vi "SetFs.vi"(8 "error in (no error)":errorcluster, 9 "Fs":dbl format="%#_6pHz", 10 "Port":string(combo), 11 "reference in":refnum<class "mmWave instrument.lvclass">) -> (0 "error out":errorcluster, 3 "reference out":refnum<class "mmWave instrument.lvclass">)   [LabVIEW 2019, in "mmWave instrument.lvclass"]
doc: "Set sampling frequency for port"
uses:
  mmWave instrument.lvclass
  mmWave HW Control/HW custom error.ctl
  mmWave HW Control/mmWave HW Control.lvlib
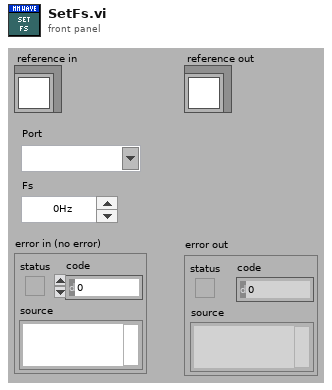
[diagram p1: front panel]
types:
  T1 = typedef "mmWave HW Control.lvlib/HW custom error.ctl" = u16
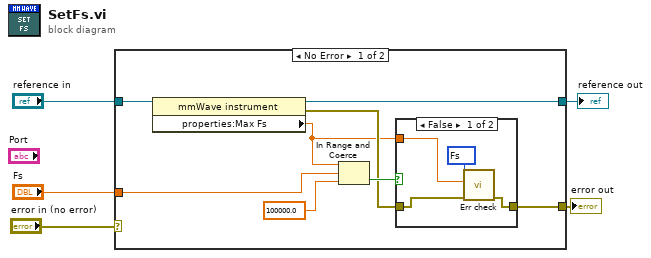
[diagram p0: block diagram]
diagram:
  n1 = case shown="No Error" "error in (no error)" {
    selector: "error in (no error)" -> [_ w20]
    tunnel: [w8 w20] -> w4
    tunnel: [w12 w19] -> w2
    tunnel: "reference in" -> [w13 w19]
    tunnel: "Fs" -> [w11 _]
    frame No Error {
      n2 = property class="mmWave instrument"(reference=w13) -> (reference out=w12:refnum<class "mmWave instrument.lvclass">, error out=w7:errorcluster, "properties:Max Fs"=w6:dbl)  [unwired: 1 in]
      n3 = In Range and Coerce(upper limit=w6, x=w11, lower limit=100000.0) -> (In Range?=w9:bool)  [unwired: 1 out]
      n4 = case shown="False" w9 {
        tunnel: [w14 w18] -> w8
        tunnel: w7 -> [w15 w18]
        tunnel: w6 -> [w17 _]
        frame False {
          w16 = T1 10003 items=["TX list"=10000, "TX length"=10001, "RX length"=10002, "Fs"=10003] ("HW custom err")
          n5 = call "Err check.vi"("error in"=w15, "Variant Control"=w17, "HW custom err"=w16) -> ("error out"=w14:errorcluster)  [unwired: 8 in]
        }
        frame True {
        }
      }
    }
    frame Error {
    }
  }
  "error out" <- w4
  "reference out" <- w2
